vi "Get Controller Variables Ranges.vi"(8 "error in (no error)":errorcluster, 10 "Path":string, 11 "NIVS.SysDef Ref":refnum<k24>) -> (0 "error out":errorcluster, 2 "Setpoint Range":cluster{"Min":dbl, "Max":dbl}, 3 "Output Range":cluster{"Min":dbl, "Max":dbl})   [LabVIEW 2019, in "Control Workspace Object.lvlib"]
uses:
  Control Workspace Object.lvlib
  NationalInstruments.VeriStand.SystemStorage
  NationalInstruments.VeriStand
  Shared/Constants.vi
  Shared/Control Addon Shared.lvlib
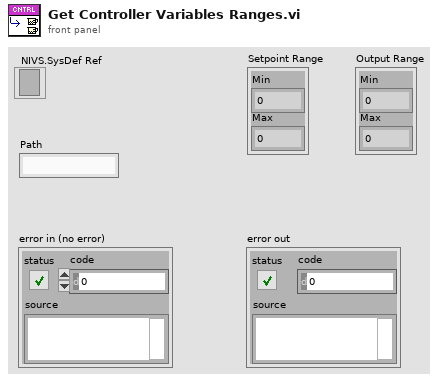
[diagram p1: front panel]
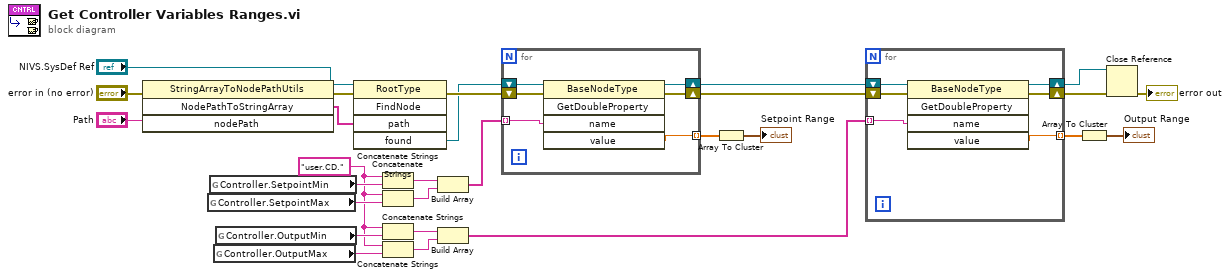
[diagram p0: block diagram]
diagram:
  w1 = "user.CD." ("string")
  n1 = invoke class="StringArrayToNodePathUtils" method="NodePathToStringArray"(error in="error in (no error)", "nodePath"="Path") -> (error out=w21:errorcluster, "NodePathToStringArray"=w23:string[])  [unwired: 2 in, 2 out]
  n2 = global read "Constants.vi" "Controller.SetpointMax"() -> (w27:string)
  n3 = global read "Constants.vi" "Controller.SetpointMin"() -> (w26:string)
  n4 = global read "Constants.vi" "Controller.OutputMax"() -> (w6:string)
  n5 = global read "Constants.vi" "Controller.OutputMin"() -> (w7:string)
  n6 = invoke class="RootType" method="FindNode"(reference="NIVS.SysDef Ref", error in=w21, "path"=w23) -> (error out=w25:errorcluster, "found"=w2:refnum<k24>)  [unwired: 2 in, 3 out]
  n7 = Concatenate Strings(w1, w26) -> (w19:string)
  n8 = Concatenate Strings(w1, w27) -> (w18:string)
  n9 = Concatenate Strings(w1, w7) -> (w8:string)
  n10 = Concatenate Strings(w1, w6) -> (w9:string)
  n11 = Build Array(w19, w18) -> (w17:string[])
  n12 = Build Array(w8, w9) -> (w5:string[])
  n13 = for {
    shift-right: [w32] -> w11
    shift-left: w2 -> [w30]
    shift-right: [w33] -> w13
    shift-left: w25 -> [w31]
    tunnel: w17 -> [w29] mode=indexing
    tunnel: [w28] -> w16 mode=indexing
    n14 = invoke class="BaseNodeType" method="GetDoubleProperty"(reference=w30, error in=w31, "name"=w29) -> (reference out=w32:refnum<k24>, error out=w33:errorcluster, "value"=w28:dbl)  [unwired: 2 in, 2 out]
  }
  n15 = Array To Cluster(array=w16) -> (cluster=→"Setpoint Range":cluster{"[0]":dbl, "[1]":dbl})
  n16 = for {
    shift-right: [w38] -> w10
    shift-left: w11 -> [w36]
    shift-right: [w39] -> w12
    shift-left: w13 -> [w37]
    tunnel: w5 -> [w35] mode=indexing
    tunnel: [w34] -> w3 mode=indexing
    n17 = invoke class="BaseNodeType" method="GetDoubleProperty"(reference=w36, error in=w37, "name"=w35) -> (reference out=w38:refnum<k24>, error out=w39:errorcluster, "value"=w34:dbl)  [unwired: 2 in, 2 out]
  }
  n18 = Array To Cluster(array=w3) -> (cluster=→"Output Range":cluster{"[0]":dbl, "[1]":dbl})
  n19 = Close Reference(reference=w10, error in (no error)=w12) -> (error out=→"error out":errorcluster)
